vi "CreateText.vi"(8 "error in (no error)":errorcluster, 10 "objName in":string, 11 "class data in":refnum<class "Text.lvclass">) -> (0 "error out":errorcluster, 3 "class data out":refnum<class "Text.lvclass">)   [LabVIEW 2010, in "Labricks.lvlib" / "Text.lvclass"]
uses:
  Text.lvclass
  <vilib>/picture/3D Picture Control/NI_3D Picture Control.lvlib
  RenderBase/SceneObject_class/SceneObject.lvclass
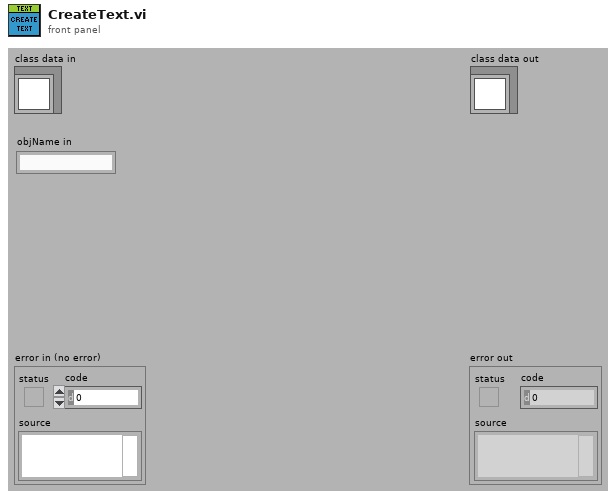
[diagram p1: front panel]
types:
  T1 = cluster{"Red":sgl, "Green":sgl, "Blue":sgl, "Alpha":sgl}
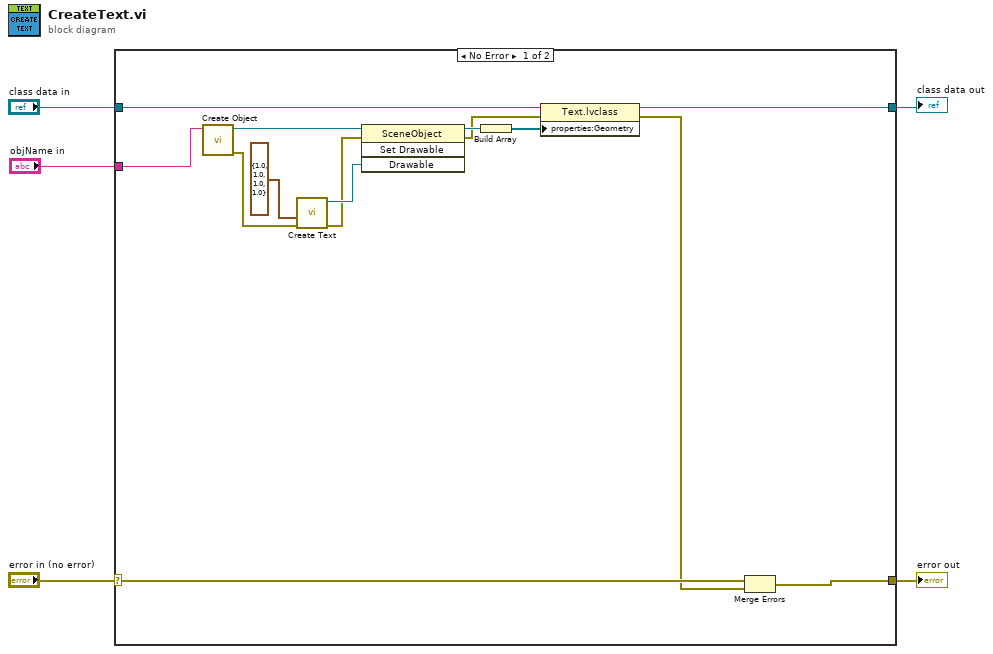
[diagram p0: block diagram]
diagram:
  n1 = case shown="No Error" "error in (no error)" {
    selector: "error in (no error)" -> [w19 w21]
    tunnel: [w7 w21] -> w4
    tunnel: "class data in" -> [w18 w20]
    tunnel: [w17 w20] -> w2
    tunnel: "objName in" -> [w11 _]
    frame No Error {
      n2 = call <vilib>:"Create Object.vi"("Name"=w11) -> ("error out"=w10:errorcluster, "Scene:New Object"=w14:refnum<vi>)  [unwired: 9 in]
      n3 = call <vilib>:"Create Text.vi"("error in (no error)"=w10, "Color"=T1 {"Red"=1.0, "Green"=1.0, "Blue"=1.0, "Alpha"=1.0}) -> ("error out"=w9:errorcluster, "New Text Refnum"=w15:refnum<vi>)  [unwired: 8 in]
      n4 = invoke class="SceneObject" method="Set Drawable"(reference=w14, error in=w9, "Drawable"=w15) -> (reference out=w12:refnum<vi>, error out=w8:errorcluster)  [unwired: 1 in, 2 out]
      n5 = Build Array(w12) -> (w16:refnum<vi>[])
      n6 = property class="Text.lvclass"(reference=w18, error in=w8, "properties:Geometry"=w16) -> (reference out=w17:refnum<class "Text.lvclass">, error out=w6:errorcluster)
      n7 = Merge Errors(w19, w6) -> (w7:errorcluster)
    }
    frame Error {
    }
  }
  "error out" <- w4
  "class data out" <- w2
